vi "Write Data To Table.vi"(2 "Cluster":T1, 3 "file path (dialog if empty)":path) -> ()   [LabVIEW 2013]
uses:
  <vilib>/Utility/file.llb/Write To Spreadsheet File (string).vi
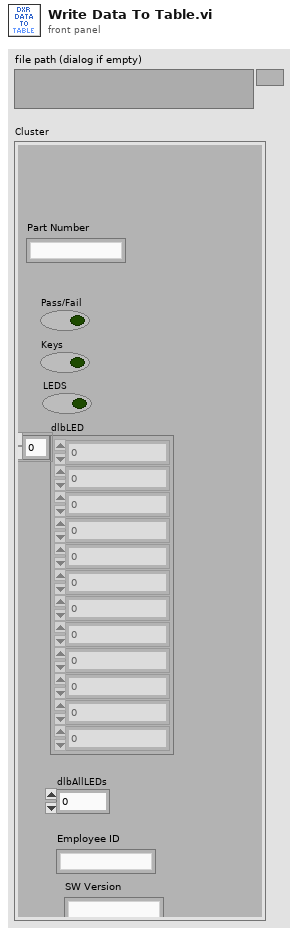
[diagram p1: front panel]
types:
  T1 = cluster{"dlbLED":dbl[], "dlbAllLEDs":dbl, "Pass/Fail":bool, "Keys":bool, "LEDS":bool, "Employee ID":string, "Part Number":string, "SW Version":string}
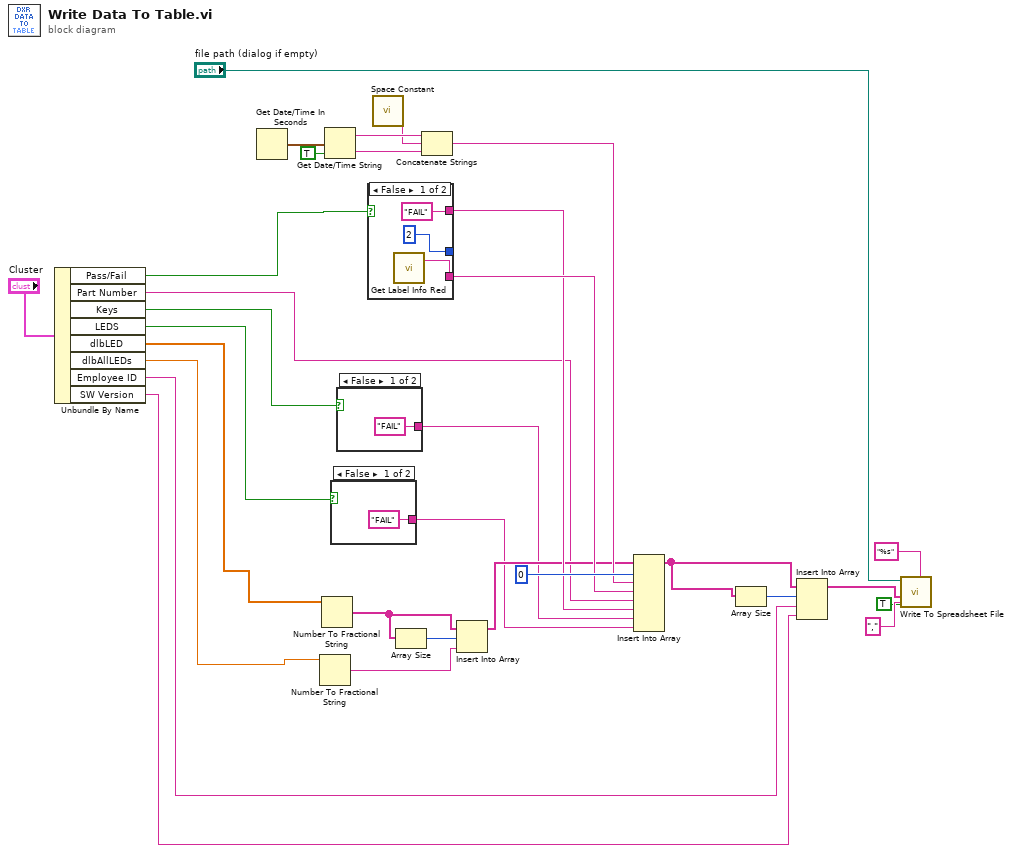
[diagram p0: block diagram]
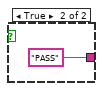
[diagram p2: hidden frame]
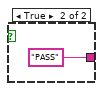
[diagram p3: hidden frame]
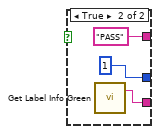
[diagram p4: hidden frame]
diagram:
  n1 = Unbundle By Name("Cluster") -> ("Pass/Fail"=w11:bool, "Part Number"=w10:string, "Keys"=w9:bool, "LEDS"=w8:bool, "dlbLED"=w7:dbl[], "dlbAllLEDs"=w6:dbl, "Employee ID"=w5:string, "SW Version"=w4:string)
  n2 = Get Date/Time In Seconds() -> (seconds since 1Jan1904=w29:timestamp)
  n3 = Number To Fractional String(number=w6) -> (F-format string=w30:string)  [unwired: 3 in]
  n4 = Number To Fractional String(number=w7) -> (F-format string=w24:string[])  [unwired: 3 in]
  n5 = Get Date/Time String(seconds (now)=w29, want seconds? (F)=TRUE) -> (date string=w27:string, time string=w26:string)  [unwired: 1 in]
  n6 = case shown="False" w8 {
    tunnel: ["FAIL" "PASS"] -> w2
    frame False {
    }
    frame True {
    }
  }
  n7 = case shown="False" w9 {
    tunnel: ["FAIL" "PASS"] -> w3
    frame False {
    }
    frame True {
    }
  }
  n8 = case shown="False" w11 {
    tunnel: [2 1] -> _
    tunnel: [w37 w40] -> w21
    tunnel: ["FAIL" "PASS"] -> w20
    frame False {
      n9 = call "Get Label Info Red.vi"() -> ("Label"=w37:string)  [unwired: 6 in]
    }
    frame True {
      n10 = call "Get Label Info Green.vi"() -> ("Label"=w40:string)  [unwired: 6 in]
    }
  }
  n11 = call <vilib>:"Space Constant.vi"() -> ("String"=w25:string)
  n12 = Array Size(array=w24) -> (size(s)=w31:i32)
  n13 = Concatenate Strings(w27, w25, w26) -> (w22:string)
  n14 = Insert Into Array(array=w24, index=w31, new element=w30) -> (w19:string[])
  n15 = Insert Into Array(array=w19, index=0, new element #1=w22, new element #2=w21, new element #3=w10, new element #4=w20, new element #5=w3, new element #6=w2) -> (w17:string[])
  n16 = Array Size(array=w17) -> (size(s)=w18:i32)
  n17 = Insert Into Array(array=w17, index=w18, new element #1=w5, new element #2=w4) -> (w14:string[])
  n18 = call-poly <vilib>:"Write To Spreadsheet File.vi"("delimiter (\\t)"="," ("delimiter (\\t)"), "format (%s)"="%s" ("format (%.3f)"), "append to file? (new file:F)"=TRUE, "1D data"=w14, "file path (dialog if empty)"="file path (dialog if empty)") -> ()  [unwired: 3 in, 1 out]
